vi "Write Camera Settings to Ini File.vi"(8 "error in (no error)":errorcluster, 10 "refnum in":T1, 11 "Camera in":refnum<class "Camera Actor.lvclass">) -> (0 "error out":errorcluster, 2 "refnum out":T1, 3 "Camera out":refnum<class "Camera Actor.lvclass">)   [LabVIEW 2014, in "Camera Actor.lvlib" / "Camera Actor.lvclass"]
uses:
  Camera Actor.lvclass
  <vilib>/Utility/config.llb/Config Data RefNum.ctl
  <vilib>/Utility/config.llb/NI_LVConfig.lvlib
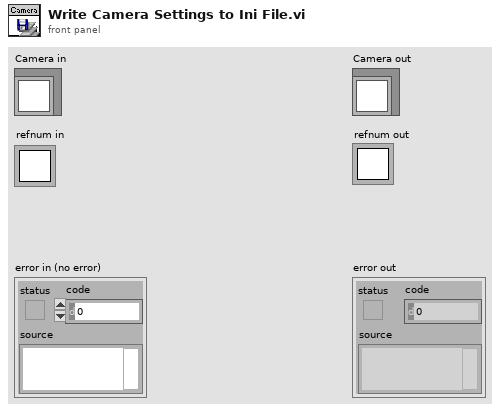
[diagram p1: front panel]
types:
  T1 = typedef "NI_LVConfig.lvlib/Config Data RefNum.ctl" = refnum<k1>
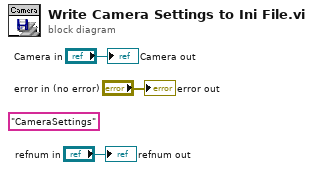
[diagram p0: block diagram]
diagram:
  (unwired) "CameraSettings"
  "error out" <- "error in (no error)"
  "Camera out" <- "Camera in"
  "refnum out" <- "refnum in"
